vi "Cleanup.vi"(8 "error in (no error)":errorcluster, 10 "System In":refnum<class "abs_System.lvclass">, 11 "Node in":refnum<class "abs_Composite.lvclass">) -> (0 "error out":errorcluster, 2 "System Out":refnum<class "abs_System.lvclass">, 3 "Node out":refnum<class "abs_Composite.lvclass">)   [LabVIEW 2021, in "BT.lvlib" / "abs_Composite.lvclass"]
uses:
  abs_Composite.lvclass
  abs_System/abs_System.lvclass
  abs_Composite.lvclass/abs_Composite.ctl
  abs_Node/abs_Node.lvclass
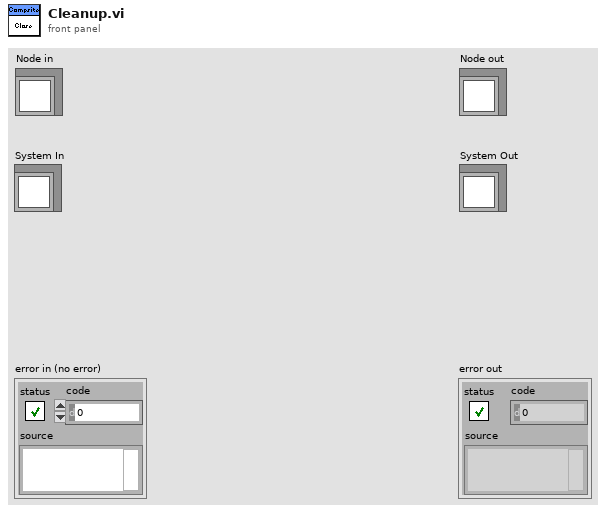
[diagram p1: front panel]
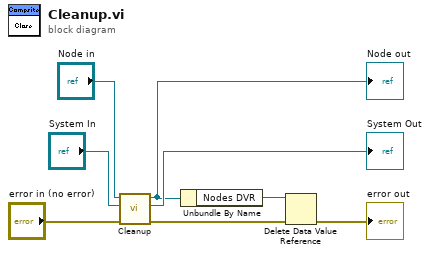
[diagram p0: block diagram]
diagram:
  n1 = call-parent "Cleanup.vi"("error in (no error)"="error in (no error)", "System In"="System In", "Node in"="Node in") -> ("error out"=w3:errorcluster, "System Out"=→"System Out":refnum<class "abs_System.lvclass">, "Node out"=w4:refnum<class "abs_Composite.lvclass">)  [unwired: 6 in]
  "Node out" <- w4
  n2 = Unbundle By Name(w4) -> ("Nodes DVR"=w2:refnum<data-value>)
  n3 = Delete Data Value Reference(data value reference=w2, error in=w3) -> (error out=→"error out":errorcluster)  [unwired: 1 out]
